vi "Peak Width.vi"(6 "Peak Y":dbl, 9 "Peak X":dbl, 10 "Y":dbl[](array[numeric]), 11 "X":dbl[](array[numeric])) -> (1 "low side":dbl, 2 "high side":dbl, 3 "width":dbl)   [LabVIEW 2016]
panel:
  out "Detected peak width":cluster{"X":dbl[], "Y":dbl[]}[](graph)
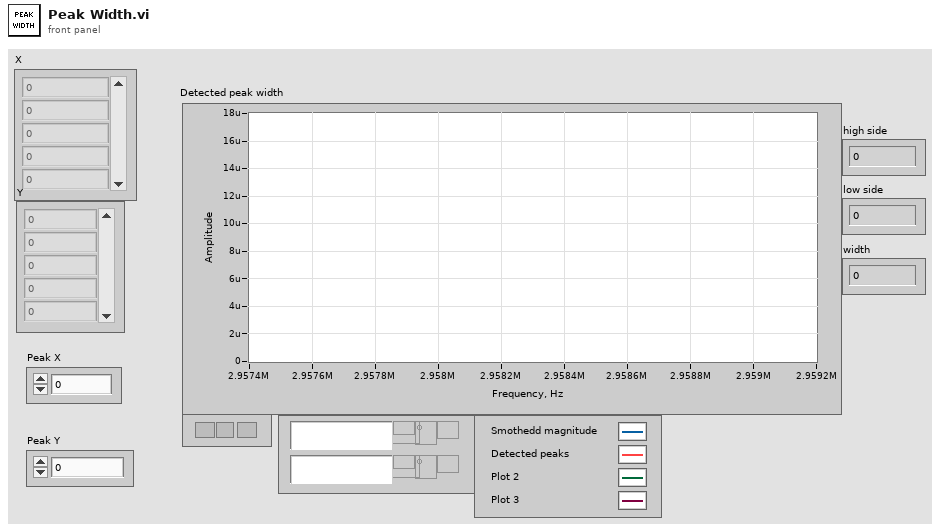
[diagram p1: front panel]
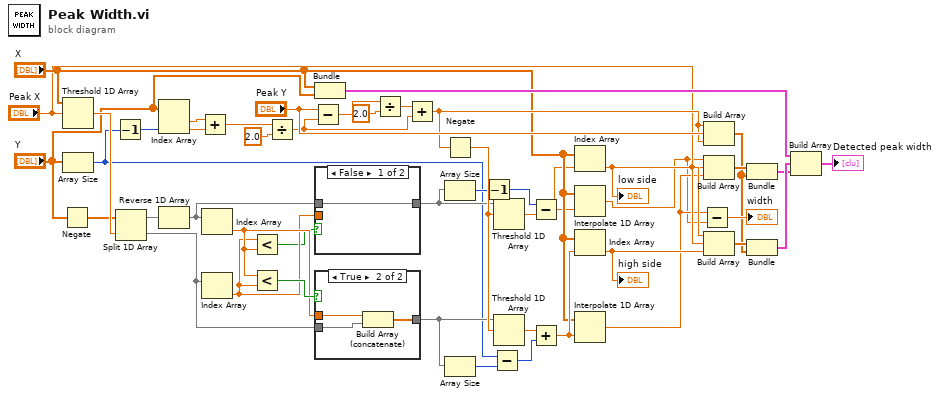
[diagram p0: block diagram]
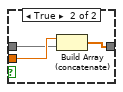
[diagram p2: hidden frame]
diagram:
  n1 = Negate(x="Y") -> (-x=w37:dbl[])
  n2 = Threshold 1D Array(2:"Peak X", 3:"X") -> (0:w44:dbl)  [unwired: 1 in]
  n3 = Array Size(array="Y") -> (size(s)=w13:i32)
  n4 = Decrement(x=w13) -> (x-1=w33:i32)
  n5 = Split 1D Array(array=w37, index=w44) -> (first subarray=w35:dbl[], second subarray=w21:dbl[])
  n6 = Index Array(array="Y", index #2=w33) -> (element #1=w32:dbl, element #2=w31:dbl)  [unwired: 1 in]
  n7 = Reverse 1D Array(array=w35) -> (reversed array=w17:dbl[])
  n8 = Add(x=w32, y=w31) -> (x+y=w30:dbl)
  n9 = Index Array(array=w17) -> (element=w20:dbl)  [unwired: 1 in]
  n10 = Index Array(array=w21) -> (element=w19:dbl)  [unwired: 1 in]
  n11 = Less?(x=w19, y=w20) -> (x < y?=w18:bool)
  n12 = Less?(x=w20, y=w19) -> (x < y?=w22:bool)
  n13 = Divide(x=w30, y=2.0) -> (x/y=w24:dbl)
  n14 = Subtract(x="Peak Y", y=w24) -> (x-y=w26:dbl)
  n15 = Bundle("X"="X", "Y"="Y") -> (w47:cluster{"X":dbl[], "Y":dbl[]})  [unwired: 1 in]
  n16 = case shown="False" w18 {
    tunnel: w19 -> [_ w51]
    tunnel: w17 -> [w48 w50]
    tunnel: [w48 w49] -> w16
    frame False {
    }
    frame True {
      n17 = Build Array (concatenate)(w51, w50) -> (w49:dbl[])
    }
  }
  n18 = case shown="True" w22 {
    tunnel: w20 -> [_ w55]
    tunnel: w21 -> [w52 w54]
    tunnel: [w52 w53] -> w15
    frame False {
    }
    frame True {
      n19 = Build Array (concatenate)(w55, w54) -> (w53:dbl[])
    }
  }
  n20 = Divide(x=w26, y=2.0) -> (x/y=w43:dbl)
  n21 = Add(x=w43, y=w24) -> (x+y=w25:dbl)
  n22 = Negate(x=w25) -> (-x=w36:dbl)
  n23 = Array Size(array=w16) -> (size(s)=w23:i32)
  n24 = Array Size(array=w15) -> (size(s)=w14:i32)
  n25 = Decrement(x=w23) -> (x-1=w1:i32)
  n26 = Subtract(x=w13, y=w14) -> (x-y=w12:i32)
  n27 = Threshold 1D Array(2:w36, 3:w16) -> (0:w34:dbl)  [unwired: 1 in]
  n28 = Threshold 1D Array(2:w36, 3:w15) -> (0:w40:dbl)  [unwired: 1 in]
  n29 = Subtract(x=w1, y=w34) -> (x-y=w9:dbl)
  n30 = Add(x=w40, y=w12) -> (x+y=w11:dbl)
  n31 = Index Array(array="X", index=w9) -> (element=w8:dbl)
  "low side" <- w8
  n32 = Interpolate 1D Array(1:w9, 2:"X") -> (0:w2:dbl)
  n33 = Index Array(array="X", index=w11) -> (element=w39:dbl)
  "high side" <- w39
  n34 = Interpolate 1D Array(1:w11, 2:"X") -> (0:w3:dbl)
  n35 = Subtract(x=w3, y=w2) -> (x-y=→"width":dbl)
  n36 = Build Array(w25, "Peak Y", w25) -> (w6:dbl[])
  n37 = Build Array(w2, "Peak X", w3) -> (w7:dbl[])
  n38 = Build Array(w8, "Peak X", w39) -> (w42:dbl[])
  n39 = Bundle(w7, w6) -> (w5:cluster{dbl[], dbl[]})  [unwired: 1 in]
  n40 = Bundle(w42, w6) -> (w41:cluster{dbl[], dbl[]})  [unwired: 1 in]
  n41 = Build Array(w47, w41, w5) -> (→"Detected peak width":cluster{"X":dbl[], "Y":dbl[]}[])
